vi "Change Map Range.vi"(5 "Current East Bounds":cluster{dbl, "Sway":dbl}, 7 "Current North Bounds":cluster{dbl, "Surge":dbl}, 8 "Range East":dbl, 9 "Range North":dbl, 10 "East":dbl, 11 "North":dbl) -> (0 "East Min":dbl, 1 "East Max":dbl format="%#_10g", 2 "North Min":dbl format="%#_10g", 3 "North Max":dbl format="%#_10g")   [LabVIEW 2014]
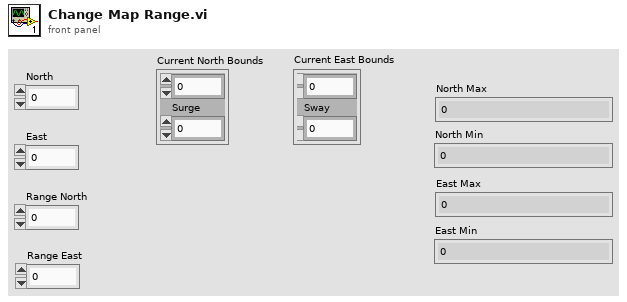
[diagram p1: front panel]
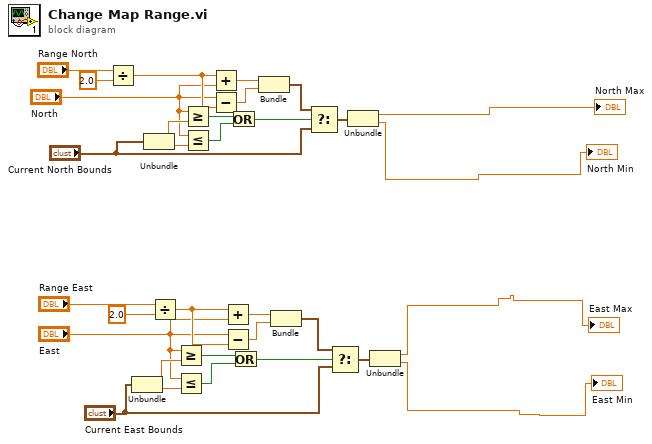
[diagram p0: block diagram]
diagram:
  n1 = Divide(x="Range North", y=2.0) -> (x/y=w22:dbl)
  n2 = Unbundle("Current East Bounds") -> (w26:dbl, "Sway"=w13:dbl)
  n3 = Unbundle("Current North Bounds") -> (w28:dbl, "Surge"=w20:dbl)
  n4 = Divide(x="Range East", y=2.0) -> (x/y=w7:dbl)
  n5 = Greater Or Equal?(x="East", y=w26) -> (x >= y?=w11:bool)
  n6 = Less Or Equal?(x="East", y=w13) -> (x <= y?=w12:bool)
  n7 = Greater Or Equal?(x="North", y=w28) -> (x >= y?=w21:bool)
  n8 = Less Or Equal?(x="North", y=w20) -> (x <= y?=w18:bool)
  n9 = Add(x=w22, y="North") -> (x+y=w32:dbl)
  n10 = Subtract(x="North", y=w22) -> (x-y=w23:dbl)
  n11 = Add(x=w7, y="East") -> (x+y=w31:dbl)
  n12 = Subtract(x="East", y=w7) -> (x-y=w5:dbl)
  n13 = Or(x=w21, y=w18) -> (x .or. y?=w17:bool)
  n14 = Or(x=w11, y=w12) -> (x .or. y?=w10:bool)
  n15 = Bundle(w32, w23) -> (w15:cluster{dbl, dbl})  [unwired: 1 in]
  n16 = Bundle(w31, w5) -> (w30:cluster{dbl, dbl})  [unwired: 1 in]
  n17 = Select(t=w15, s=w17, f="Current North Bounds") -> (s? t:f=w14:cluster{dbl, "Surge":dbl})
  n18 = Select(t=w30, s=w10, f="Current East Bounds") -> (s? t:f=w29:cluster{dbl, "Sway":dbl})
  n19 = Unbundle(w14) -> (→"North Max":dbl, "Surge"=→"North Min":dbl)
  n20 = Unbundle(w29) -> (→"East Max":dbl, "Sway"=→"East Min":dbl)
